vi "Questionable Data Status.vi"(7 "Set/Check? (F:Set)":bool, 8 "error in (no error)":errorcluster, 9 "Check Register(0:Cond)":enum16{"Condition", "Enable", "Event"}(ring), 10 "Enable Value (0)":u16, 11 "VISA Resource Name":refnum<visa-resource-name>) -> (0 "error out":errorcluster, 2 "Bits Set":bool[](array[boolean]), 3 "VISA Resource Name Out":refnum<visa-resource-name>)   [LabVIEW 2012, in "Agilent 34970.lvlib"]
doc: "This VI allows you to set or check the Questionable Data Status registers."
uses:
  <instrlib>/Agilent 34970/Agilent 34970.lvlib
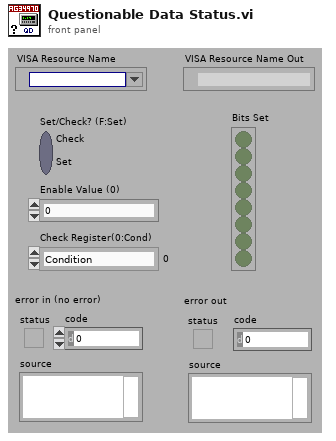
[diagram p1: front panel]
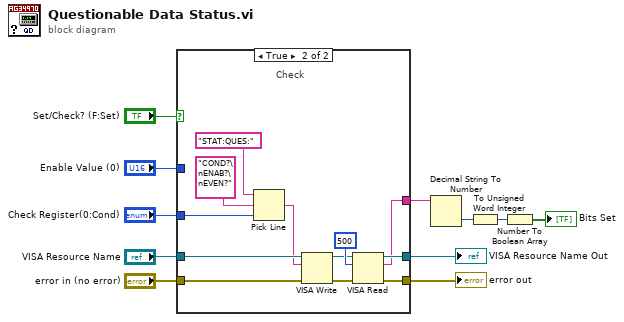
[diagram p0: block diagram]
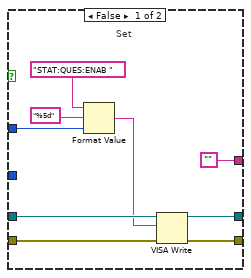
[diagram p2: hidden frame]
diagram:
  n1 = case shown="True" "Set/Check? (F:Set)" {
    tunnel: "Enable Value (0)" -> [w19 _]
    tunnel: "VISA Resource Name" -> [w18 w30]
    tunnel: "error in (no error)" -> [w17 w29]
    tunnel: [w16 w23] -> w2
    tunnel: [w15 w24] -> w3
    tunnel: "Check Register(0:Cond)" -> [_ w28]
    tunnel: ["" w22] -> w8
    frame False {
      # "Set"
      n2 = Format Value(string ("")="STAT:QUES:ENAB ", format string="%5d", value (0)=w19) -> (output string=w12:string)
      n3 = VISA Write(VISA resource name=w18, write buffer=w12, error in (no error)=w17) -> (VISA resource name out=w16:refnum<visa-resource-name>, error out=w15:errorcluster)  [unwired: 1 out]
    }
    frame True {
      # "Check"
      n4 = Pick Line(string ("")="STAT:QUES:", multi-line string="COND?\nENAB?\nEVEN?", line index=w28) -> (output string=w21:string)
      n5 = VISA Write(VISA resource name=w30, write buffer=w21, error in (no error)=w29) -> (VISA resource name out=w26:refnum<visa-resource-name>, error out=w25:errorcluster)  [unwired: 1 out]
      n6 = VISA Read(VISA resource name=w26, byte count=u32 500 ("byte count (0)"), error in (no error)=w25) -> (VISA resource name out=w23:refnum<visa-resource-name>, read buffer=w22:string, error out=w24:errorcluster)  [unwired: 1 out]
    }
  }
  "error out" <- w3
  "VISA Resource Name Out" <- w2
  n7 = Decimal String To Number(string=w8) -> (number=w7:i32)  [unwired: 2 in, 1 out]
  n8 = To Unsigned Word Integer(number=w7) -> (unsigned 16bit integer=w6:u16)
  n9 = Number To Boolean Array(number=w6) -> (Boolean array=→"Bits Set":bool[])
